vi "地块可否扩展.vi"(2 "索引":i32, 3 "地图":i16[][](array[numeric])) -> (0 "输出地图":i16[][](array[numeric]), 1 "可展开":bool)   [LabVIEW 2017]
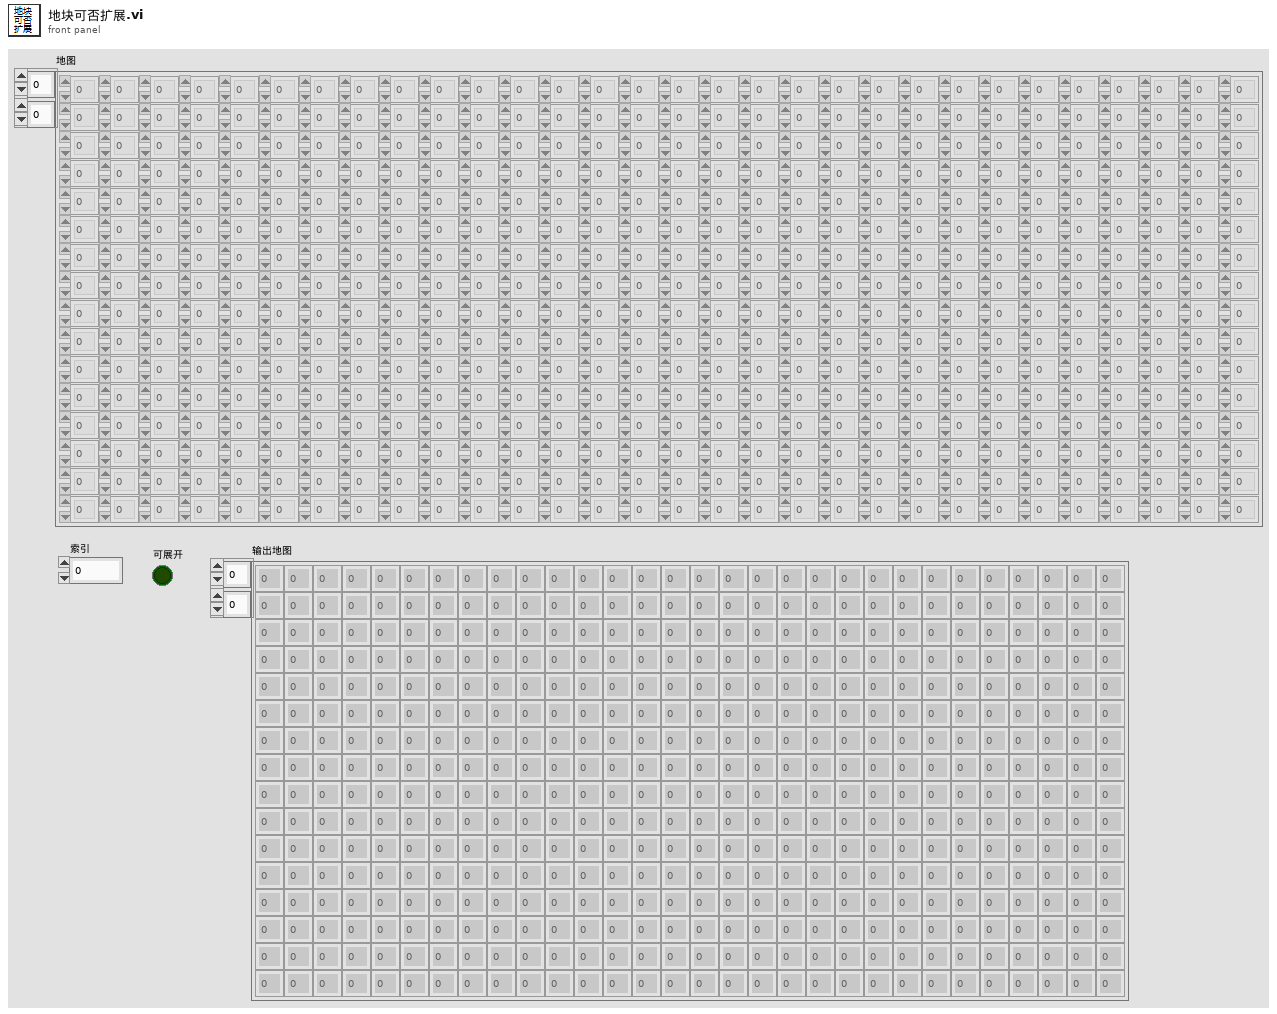
[diagram p1: front panel]
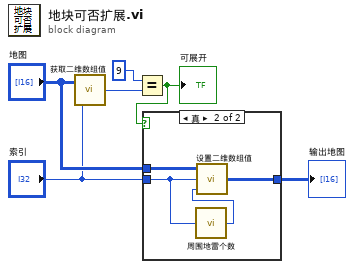
[diagram p0: block diagram]
diagram:
  n1 = call "获取二维数组值.vi"("索引"="索引", "数组"="地图") -> ("数值"=w6:i32)
  n2 = Equal?(x=9, y=w6) -> (x = y?=w4:bool)
  "可展开" <- w4
  n3 = case shown="真" w4 {
    tunnel: "地图" -> [w7 w11]
    tunnel: "索引" -> [_ w9]
    tunnel: [w7 w8] -> w1
    frame False {
    }
    frame True {
      n4 = call "周围地雷个数.vi"("索引"=w9) -> ("数值"=w10:i32)
      n5 = call "设置二维数组值.vi"("数值"=w10, "索引"=w9, "数组"=w11) -> ("输出数组"=w8:i32[][])
    }
  }
  "输出地图" <- w1
